vi "NI 5772 (AC) - Digitizer_v1.2 (FPGA).vi"() -> ()   [LabVIEW 2020]
doc: "Example Description:\nThis example demonstrates how to enable Time Interleaved Sampling with the NI 5772 adapter module to achieve a sampling rate of 1.6GS/s. This example continuously acquires records of analog input data from the NI 5772 adapter module. It allows you to select an AI channel, trigger type, and record size. This VI must be compiled before it is run. \n\nRunning the VI:\nThis VI must be run from the NI 5772 - Getting Started (Host).vi. Refer to the host VI documentation for steps regarding running and configuring the FPGA VI. \n\nExecution Steps:\nRefer to the Block Diagram of this VI for execution comments."
uses:
  Controls/AI Trigger Type.ctl
  Controls/Aquire State.ctl
  <vilib>/Platform/TimedLoop/XDataNode/timing_clust.ctl
  <vilib>/Platform/TimedLoop/XDataNode/nitl_modes.ctl
  <vilib>/Platform/TimedLoop/XDataNode/wakeup.ctl
  Controls/DigitizerState.ctl
  <vilib>/rvi/Emulation/niFpgaGetClockAttributes.vi
  <vilib>/rvi/Emulation/niFpgaSctlEmulationGetInTimedLoop.vi
  <vilib>/rvi/Emulation/niFpgaEmulationReportErrorSimple.vi
  <vilib>/rvi/eio/common/nirviEmuTemplateMethod_errors.vi
  <vilib>/rvi/Emulation/niFpgaCriticalErrorInLSC.vi
  <vilib>/rvi/Emulation/niFpgaProcessEmulError.vi
  <vilib>/rvi/Emulation/niFpgaEmulationIsFPGAContextNoSignature.vi
  <vilib>/rvi/errors/niFpgaSetErrorForExecOnDevCompSimple.vi
  <vilib>/rvi/eio/common/nirviEmuReportErrorAndStop.vi
  <vilib>/rvi/DataTransferAndStorage/Container/Common/niFpgaContainerGetUniqueNameForEmu.vi
  <vilib>/rvi/FIFO/Fifo_Resource/nirvififoEmulationSetSize.vi
  <vilib>/rvi/FIFO/Fifo_Resource/nirviFifoEmulationQueueMgr.vi
  <instcachedir>/0/nirviFifoEmulationQueueMgr_E5CAEC123FF24DC58D834DCA3CDAA9B5.lvgen/nirviFifoEmulationQueueMgr_E5CAEC123FF24DC58D834DCA3CDAA9B5_004.vi
  <vilib>/Utility/error.llb/Clear Errors.vi
  <vilib>/rvi/FIFO/Fifo_Resource/nirvififoEmulationCreateLock.vi
  <vilib>/rvi/FIFO/Fifo_Resource/nirvififoEmulationObtainLock.vi
  <vilib>/rvi/FIFO/Fifo_Resource/nirvififoEmulationReleaseLock.vi
  <vilib>/rvi/occurrence/nirviWaitOnOccurrenceBase.vi
  <vilib>/rvi/errors/nirviReportUnexpectedCaseInternalError.vi
  <vilib>/rvi/errors/nirviReportUnexpectedCaseInternalError (U32).vi
  <vilib>/rvi/Memory/Memory_Emulation/nirvimemoryFastEmulation.vi
  <vilib>/rvi/Memory/Memory_Emulation/nirvimemoryEmulation.vi
  <instcachedir>/0/nirviFifoEmulationQueueMgr_E5CAEC123FF24DC58D834DCA3CDAA9B5.lvgen/nirviFifoEmulationQueueMgr_E5CAEC123FF24DC58D834DCA3CDAA9B5_000.vi
  <vilib>/rvi/interface/RandomDataEmulation/niFpgaRandomDataHandleErrors.vi
  <vilib>/rvi/FIFO/Fifo_Resource/nirvififoEmulationDetermineInputValidOut.vi
  <instrlib>/_niInstr/Basic Elements/v1/FPGA/Private/Count Up U64.vi
  <vilib>/eio/EIONode/EIONode.xnode
  <vilib>/rvi/DataTransferAndStorage/Container/XNode/niFpgaContainer.xnode
  <vilib>/rvi/FIFO/Fifo_Resource/nirvififoEmulationRead.vi
  <vilib>/Platform/TimedLoop/XDataNode/XDataNode.xnode
  <vilib>/rvi/interface/RandomDataEmulation/nirviRandomDataFpgaReadWriteTemplate.vi
  <vilib>/rvi/FIFO/Fifo_Resource/nirvififoEmulationWrite.vi
  <vilib>/Platform/TimedLoop/XDataNode/XDNodeRunTimeDep.lvlib
  <instrlib>/_niInstr/Basic Elements/v1/FPGA/niInstr Basic Elements v1 FPGA.lvlib
  <vilib>/rvi/FIFO/Fifo_Resource/nirvififoEmulationGetNumberOfElementsToRead.vi
panel:
  out "WaitForWave\nCompletion":u16
  in  "Wave Sampling Rate":sgl
  in  "WaveSampleCount":sgl format="%#_13g"
  in  "Delay (us)":sgl
  in  "AvgCount_powerOf2":i16=1
  out "DMA FIFO Overflow?":bool caption="FIFO Overflow?"
  out "Removed\nElement":u64
  out "AvgCount":u16=1
  in  "vi/nGenTrig":bool
  in  "TrigIn Simulate":bool
  out "Trig Count":u64
  in  "Clear Count":bool
  out "Delay after Trig [cycles]":u16
  out "TS FIFO In Overflow?":bool caption="FIFO Overflow?"
  in  "Samples Per Trigger":u16=512 min=1 step=1
  in  "Arm Trigger":bool
  in  "User Command Commit":bool
  in  "User Command":u8
  out "User Command Idle":bool
  out "User Command Status":u8
  in  "User Data 0":u16
  in  "User Data 1":u8
  out "PLL Locked":bool
  out "User Error":bool
  out "Configured?":bool
  in  "Trigger Level":i16
  in  "Trigger Type":T1
  # "Resource Configuration"
  # "Analog Input"
  # "Clock Configuration"
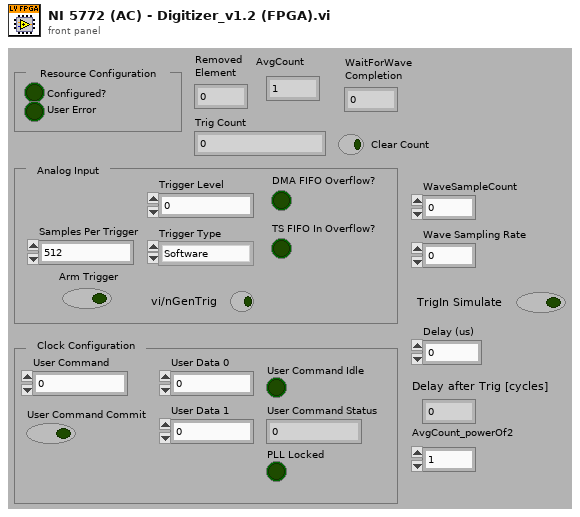
[diagram p1: front panel]
types:
  T1 = typedef "AI Trigger Type.ctl" = enum8{"Software", "Data Edge"}
  T2 = typedef "DigitizerState.ctl" = enum16{"Init", "Build/Clear Accumulator", "GetData", "AverageCountCheck", "SendtoHost"}
  T3 = typedef "Aquire State.ctl" = enum8{"Idle", "Wait for Trigger", "Hold Aquire", "Acquire", "WaitForWaveCompletion", "CheckAvg"}
  T4 = typedef "XDNodeRunTimeDep.lvlib/timing_clust.ctl" = cluster{"Expected End [f-1]":u64, "Actual End [f-1]":u64, "Finished Late? [f-1]":bool, "Expected End [i-1]":u64, "Actual End [i-1]":u64, "Finished Late? [i-1]":bool, "Expected Start [i]":u64, "Actual Start [i]":u64, "Expected Start [f]":u64, "Actual Start [f]":u64, "Source Name":string, "Structure Name":string, "Period":i64, "Deadline":i64, "Offset":i64, "Start":i64, "Priority":i32, "Timeout":i32, "Mode":T5, "Wakeup Reason":T6, "Error":errorcluster, "Source Type":string, "Secondary Source Type":string, "Global End Time":u64, "Global Start Time":u64, "Frame Duration":u64, "Iteration Duration":u64, "Assigned CPU":i32, "I/O Scan Engine Mode":u32}
  T5 = typedef "XDNodeRunTimeDep.lvlib/nitl_modes.ctl" = enum32{"No Change", "Process missed periods, maintain original phase", "Discard missed periods, maintain original phase", "Process missed periods, ignore original phase", "Discard missed periods, ignore original phase"}
  T6 = typedef "XDNodeRunTimeDep.lvlib/wakeup.ctl" = enum32{"Normal", "Aborted", "Asynchronous wakeup", "Timing source error", "Timed loop error", "Timeout"}
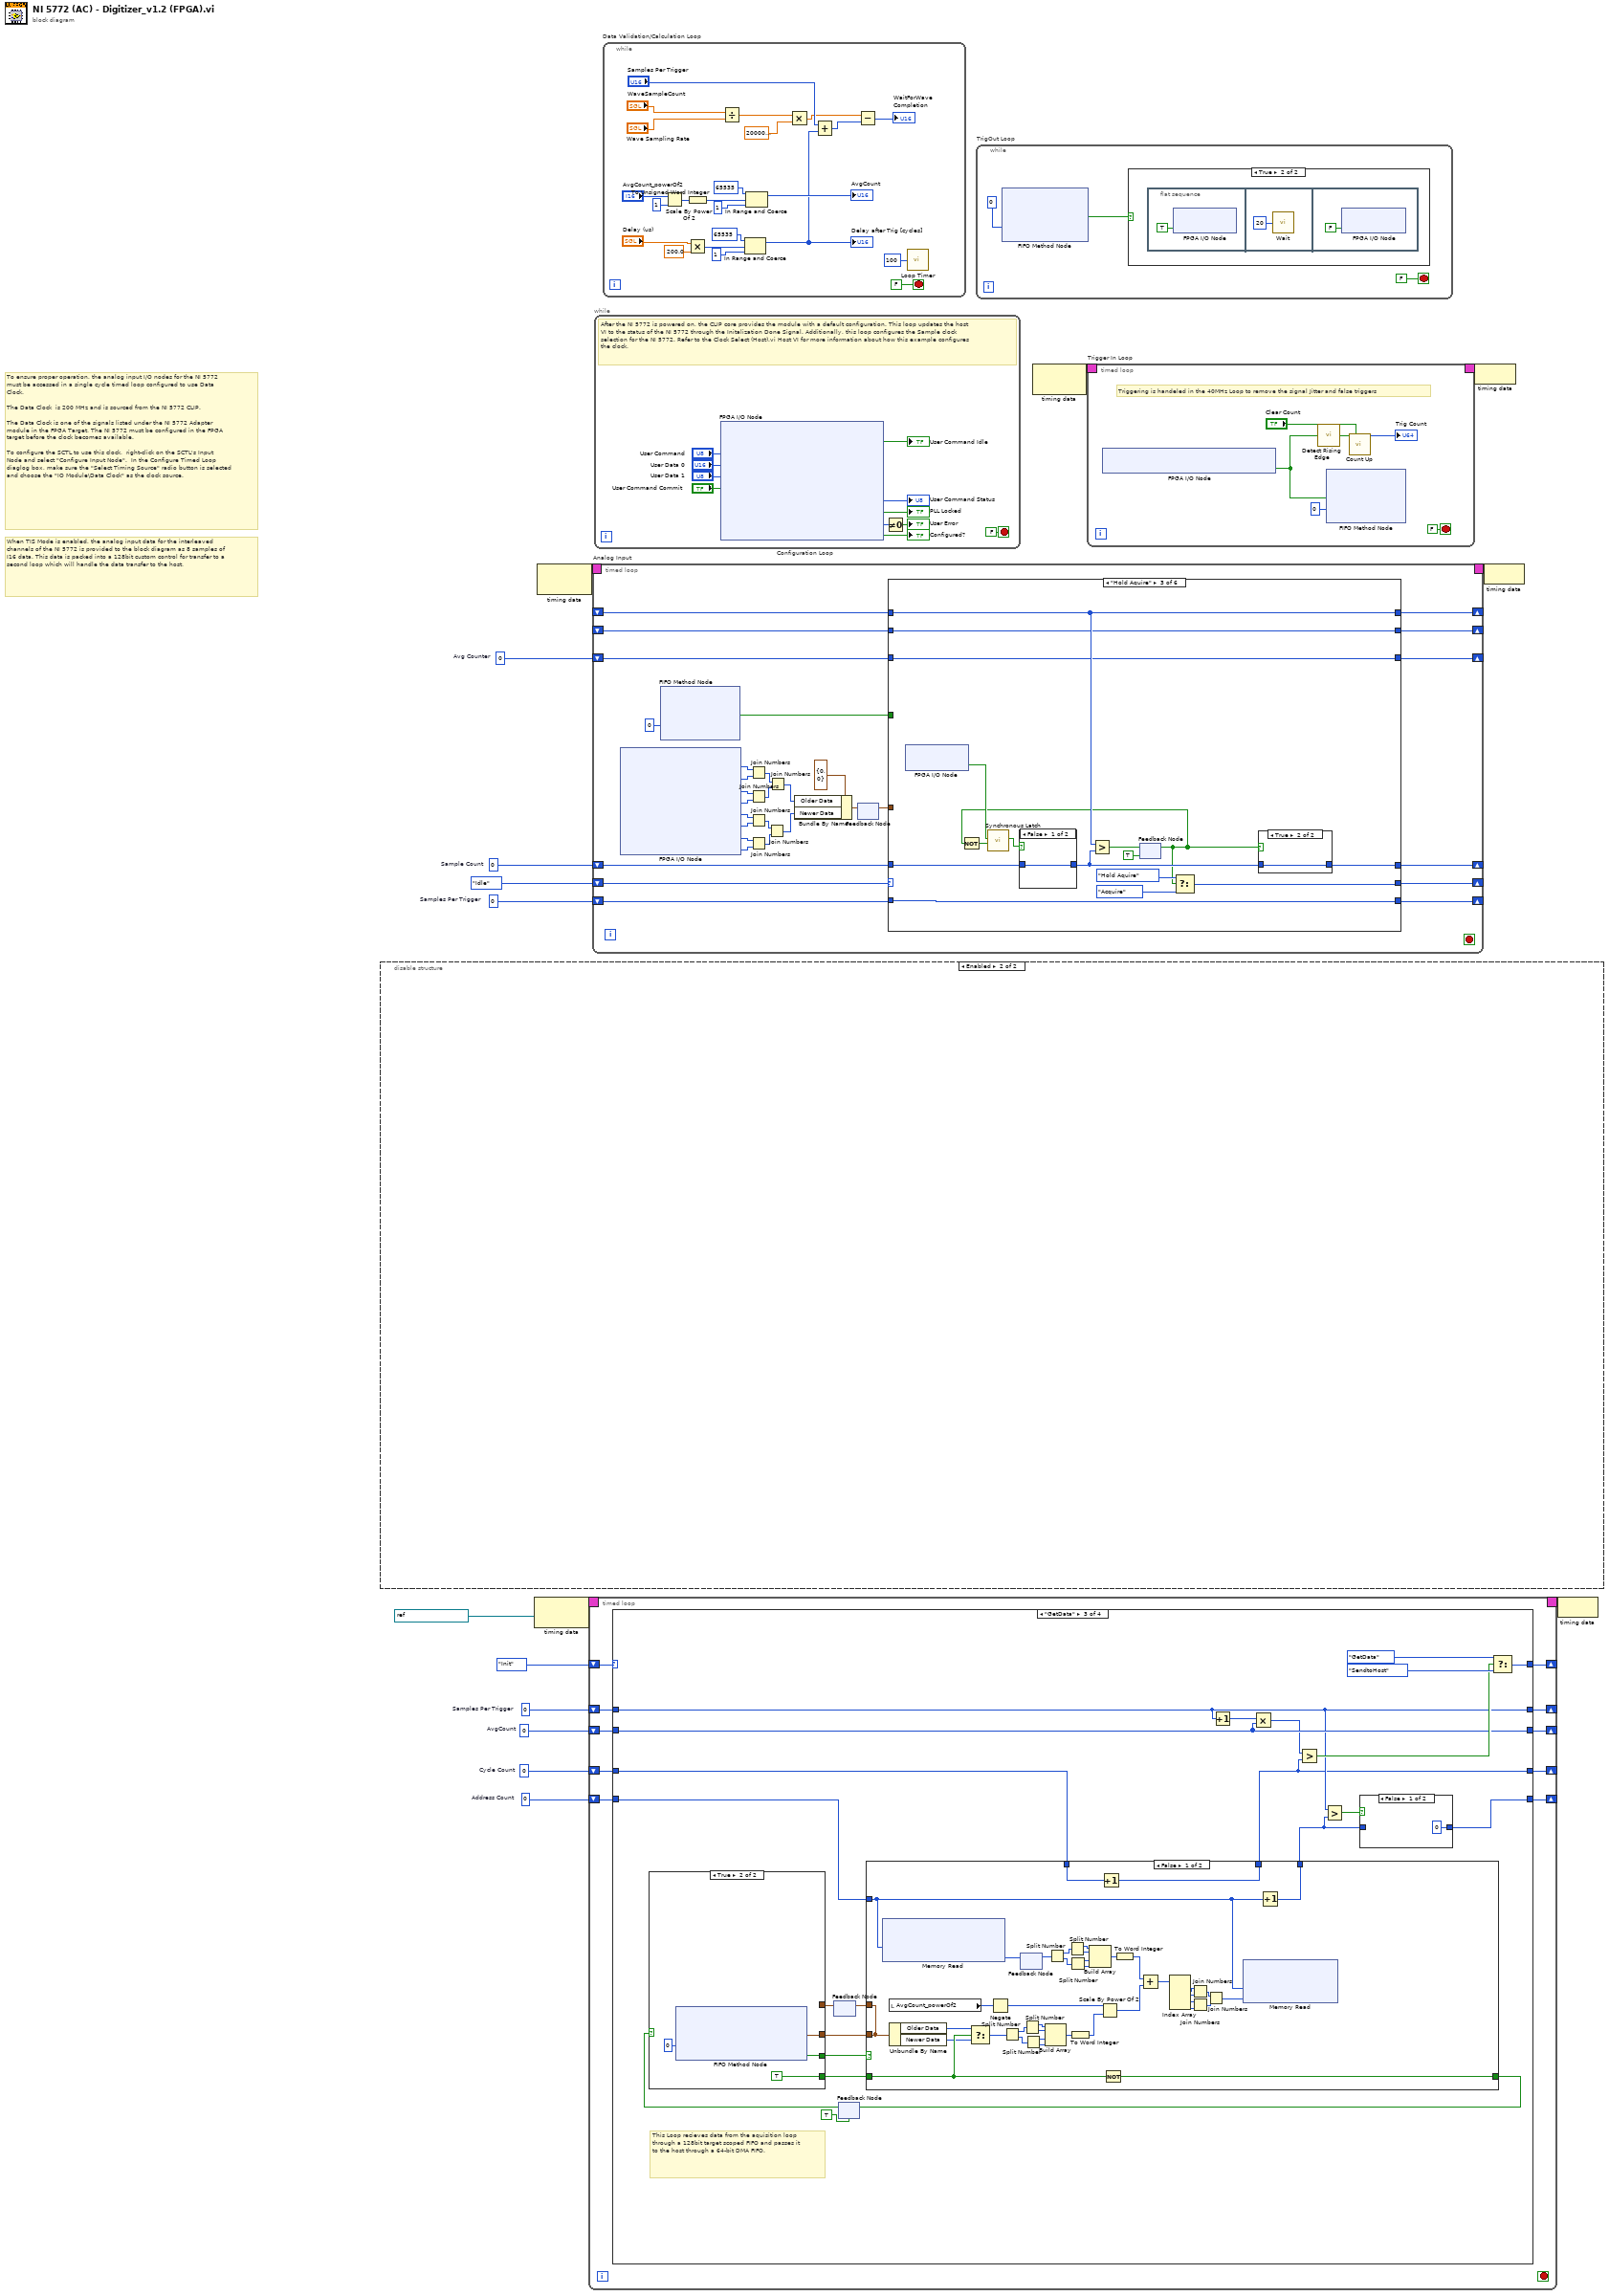
[diagram p0: block diagram]
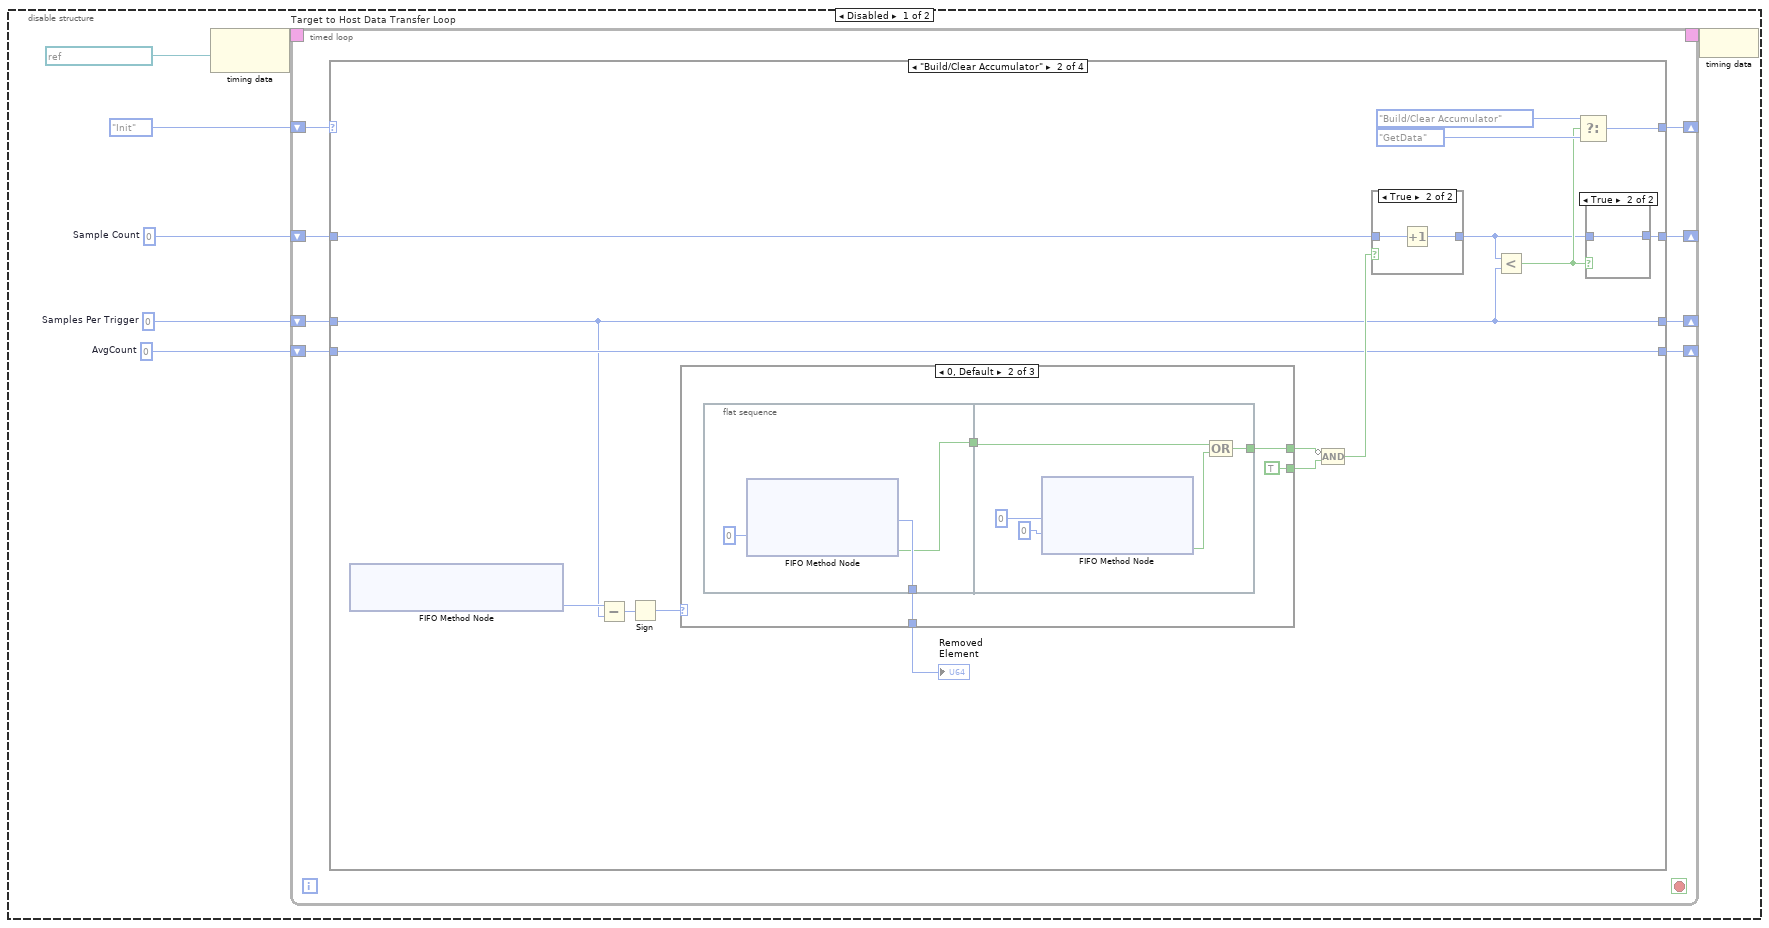
[diagram p2: hidden frame]
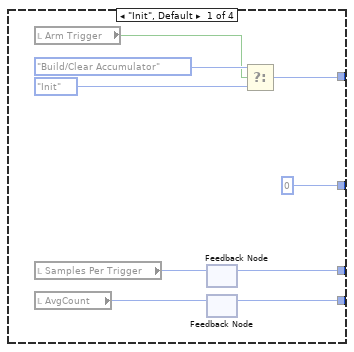
[diagram p3: hidden frame]
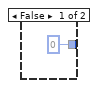
[diagram p4: hidden frame]
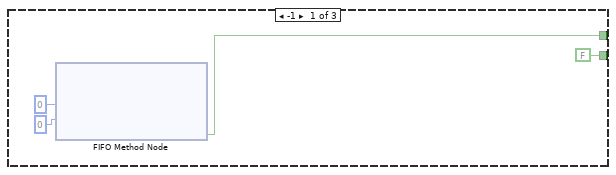
[diagram p6: hidden frame]
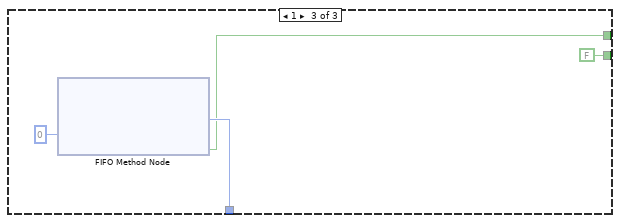
[diagram p7: hidden frame]
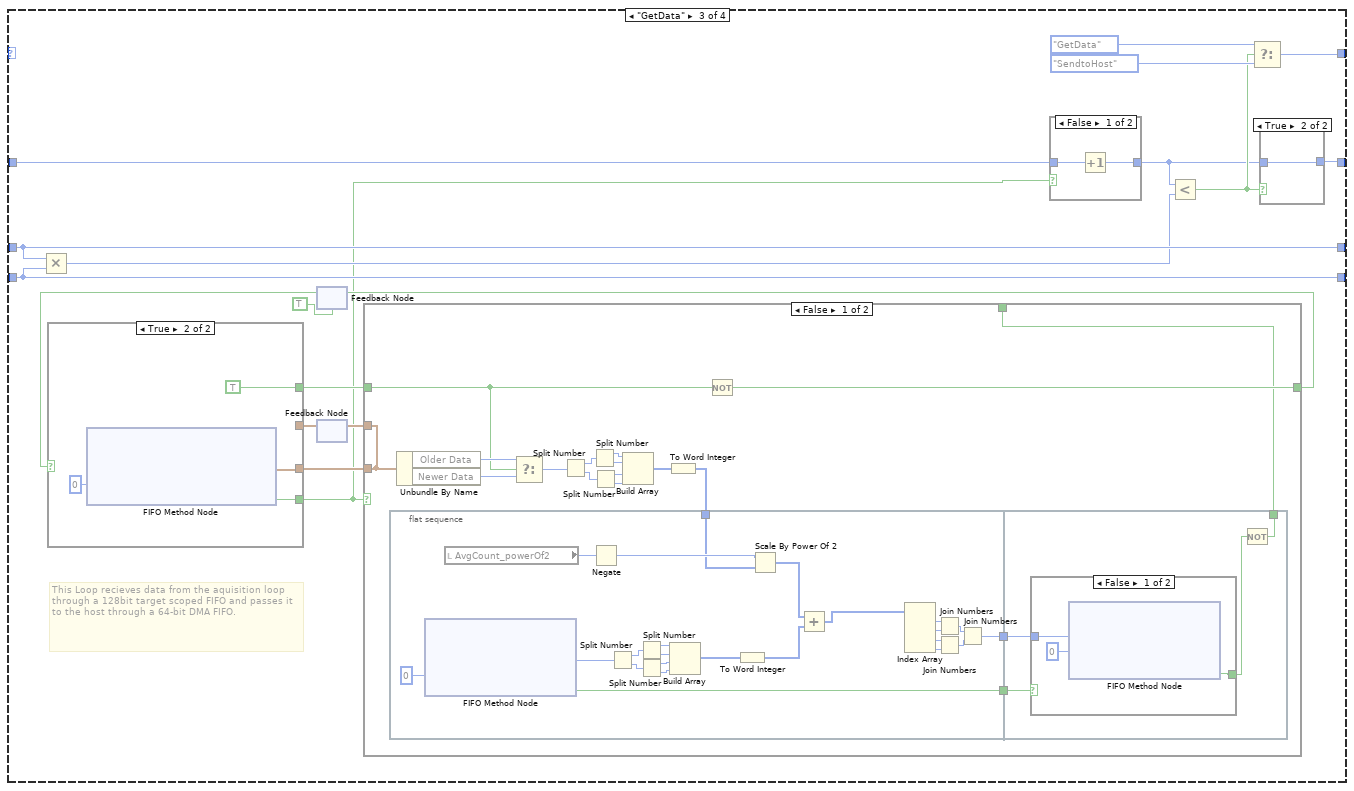
[diagram p8: hidden frame]
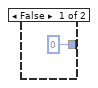
[diagram p9: hidden frame]
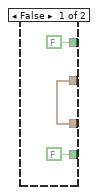
[diagram p11: hidden frame]
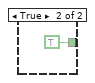
[diagram p12: hidden frame]
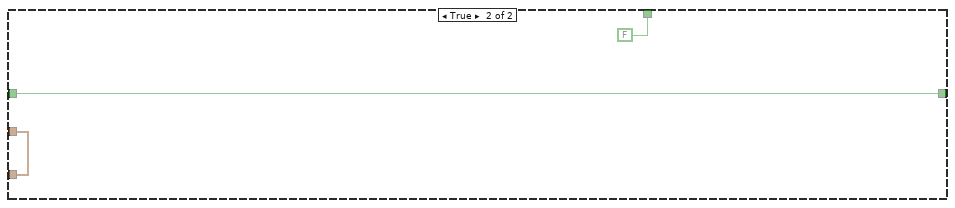
[diagram p13: hidden frame]
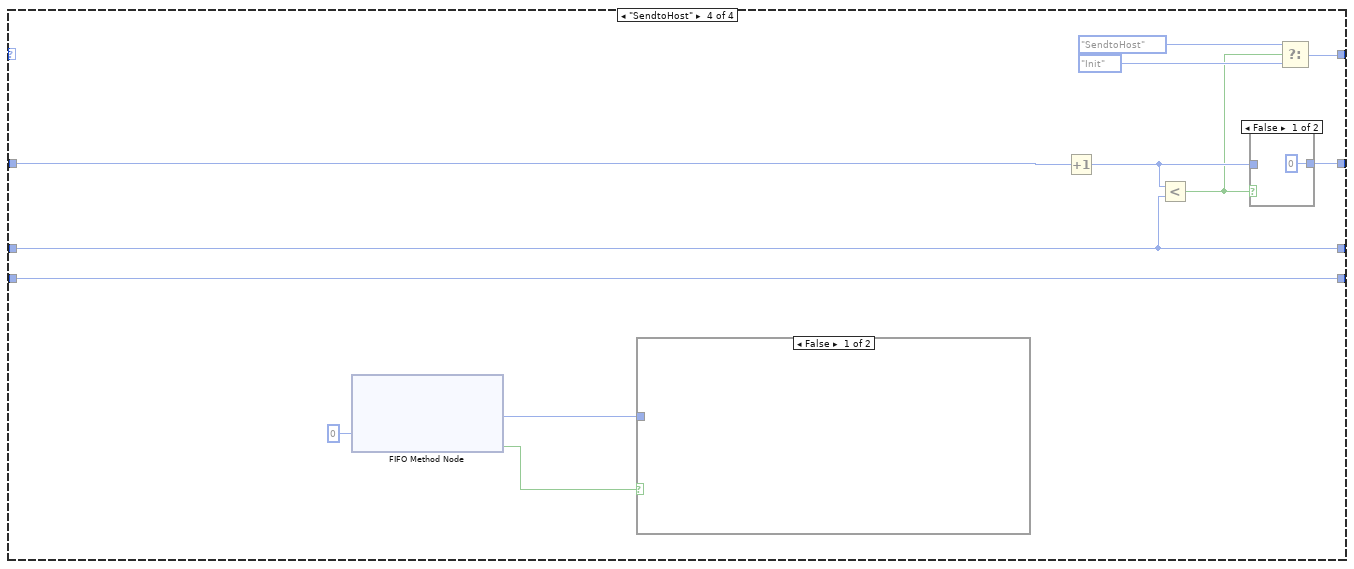
[diagram p14: hidden frame]
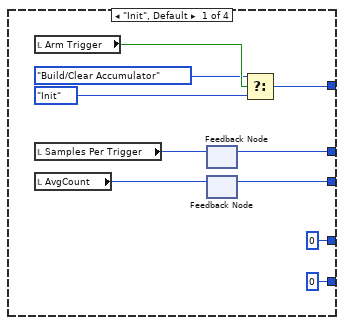
[diagram p17: hidden frame]
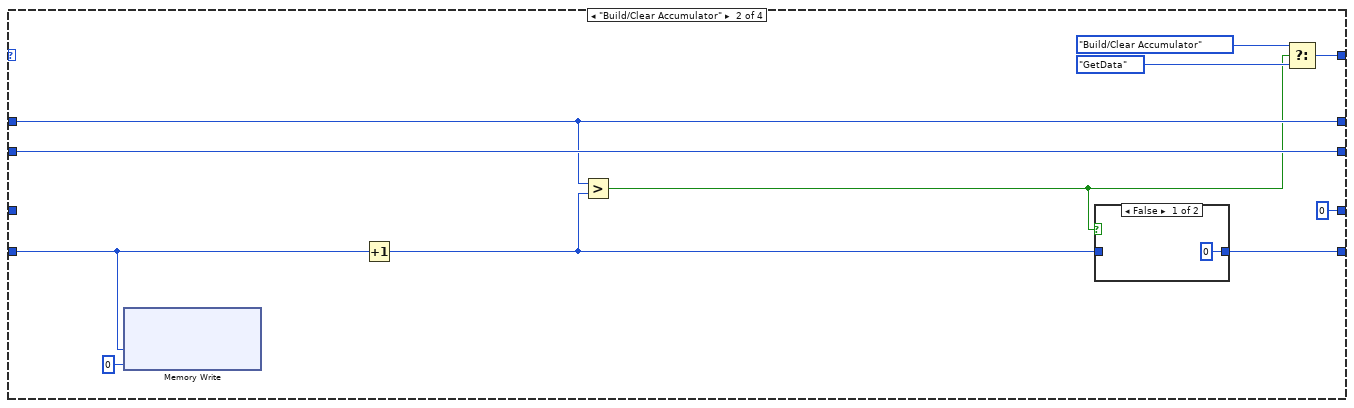
[diagram p18: hidden frame]
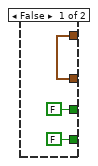
[diagram p20: hidden frame]
diagram:
  w1 = u32 0  # Cycle Count
  w2 = u32 0  # Address Count
  w3 = u16 0  # AvgCount
  w4 = u16 0  # Samples Per Trigger
  w9 = u16 0  # Avg Counter
  w12 = u16 0  # Samples Per Trigger
  w13 = u16 0  # Sample Count
  # "When TIS Mode is enabled, the analog input data for the interleaved channels of the NI 5772 is provided to the block diagram as 8 samples of I16 data. This data is packed into a 128bit custom control for transfer to a second loop which will handle the data transfer to the host."
  # "To ensure proper operation, the analog input I/O nodes for the NI 5772 must be accessed in a single cycle timed loop configured to use Data Clock. \n\nThe Data Clock  is 200 MHz and is sourced from the NI 5772 CLIP.\n\nThe Data Clock is one of the signals listed under the NI 5772 Adapter module in the FPGA Target. The NI 5772 must be configured in the FPGA target before the clock becomes available. \n\nTo configure the SCTL to use this clock,  right-click on the SCTL's Input Node and select \"Configure Input Node\".  In the Configure Timed Loop diaglog box, make sure the \"Select Timing Source\" radio button is selected and choose the \"IO Module\\Data Clock\" as the clock source."
  n1 = disable-structure shown="Enabled" {
    frame Disabled {
      w17 = u16 0  # Sample Count
      w18 = u16 0  # Samples Per Trigger
      w19 = u16 0  # AvgCount
      n2 = node-c288(refnum<k21> "100 MHz Clock" ("Source Name")) -> (w23:T4)
      n3 = timed-loop "Target to Host Data Transfer Loop" {
        timing: w23 -> [_]
        timing-out: [_] -> w22
        shift-right: [w26] -> _
        shift-left: DigitizerState."Init" -> [w31]
        shift-right: [w30] -> _
        shift-left: w18 -> [w29]
        shift-right: [w28] -> _
        shift-left: w19 -> [w27]
        shift-right: [w24] -> _
        shift-left: w17 -> [w25]
        stop <- _ stop-if-true
        n4 = case shown="\"Build/Clear Accumulator\"" w31 {
          tunnel: [w39 w44 w92 w166] -> w30
          tunnel: w29 -> [_ w44 w92 w166]
          tunnel: [w37 w45 w91 w173] -> w28
          tunnel: w27 -> [_ w45 w91 w173]
          tunnel: [w33 w52 w86 w169] -> w26
          tunnel: w25 -> [_ w47 w85 w167]
          tunnel: [u16 0 ("Sample Count") w41 w84 w164] -> w24
          frame "Init", Default {
            n5 = local read "Arm Trigger"() -> (w34:bool)
            n6 = local read "Samples Per Trigger"() -> (w40:u16)
            n7 = local read "AvgCount"() -> (w38:u16)
            n8 = feedback #1() -> (w39:u16)  [unwired: 1 in]
            n9 = feedback-in #1(w40) -> ()
            n10 = feedback #2() -> (w37:u16)  [unwired: 1 in]
            n11 = feedback-in #2(w38) -> ()
            n12 = Select(t=DigitizerState."Build/Clear Accumulator", s=w34, f=DigitizerState."Init") -> (s? t:f=w33:T2)
          }
          frame "Build/Clear Accumulator" {
            n13 = xnode ("FIFO Method Node")() -> ("Number of Elements to Read"=w56:u32)  [unwired: 1 in, 1 out]
            n14 = Subtract(x=w56, y=w44) -> (x-y=w55:i8)
            n15 = Sign(1:w55) -> (0:w54:i8)
            n16 = case shown="0, Default" w54 {
              tunnel: [_ w69 w80] -> w53
              tunnel: [w63 w67 w79] -> w49
              tunnel: [FALSE TRUE FALSE] -> w48
              frame -1 {
                n17 = xnode ("FIFO Method Node")("Element"=u64 0, "Timeout"=0) -> ("Timed Out?"=w63:bool)  [unwired: 1 in, 1 out]
              }
              frame 0, Default {
                n18 = flat-sequence {
                  tunnel: [w71] -> w69
                  tunnel: [w70] -> w68
                  tunnel: w68 -> [w75]
                  tunnel: [w73] -> w67
                  frame #0 {
                    n19 = xnode ("FIFO Method Node")("Timeout"=0) -> ("Element"=w71:u64, "Timed Out?"=w70:bool)  [unwired: 1 in, 1 out]
                  }
                  frame #1 {
                    n20 = xnode ("FIFO Method Node")("Element"=u64 0 ("y"), "Timeout"=0) -> ("Timed Out?"=w74:bool)  [unwired: 1 in, 1 out]
                    n21 = Compound Arithmetic op=OR(w75, w74) -> (w73:bool)
                  }
                }
              }
              frame 1 {
                n22 = xnode ("FIFO Method Node")("Timeout"=0) -> ("Element"=w80:u64, "Timed Out?"=w79:bool)  [unwired: 1 in, 1 out]
              }
            }
            "Removed\nElement" <- w53
            n23 = Compound Arithmetic op=AND(invert w49, w48) -> (w46:bool)
            n24 = case shown="True" w46 {
              tunnel: w47 -> [w59 w61]
              tunnel: [w59 w60] -> w42
              frame False {
              }
              frame True {
                n25 = Increment(x=w61) -> (x+1=w60:u16)
              }
            }
            n26 = Less?(x=w42, y=w44) -> (x < y?=w43:bool)
            n27 = Select(t=DigitizerState."Build/Clear Accumulator", s=w43, f=DigitizerState."GetData") -> (s? t:f=w52:T2)
            n28 = case shown="True" w43 {
              tunnel: [u16 0 ("Sample Count") w58] -> w41
              tunnel: w42 -> [_ w58]
              frame False {
              }
              frame True {
              }
            }
          }
          frame "GetData" {
            # "This Loop recieves data from the aquisition loop through a 128bit target scoped FIFO and passes it to the host through a 64-bit DMA FIFO."
            n29 = Multiply(x=w92, y=w91) -> (x*y=w83:u16)
            n30 = feedback #3(TRUE ("Timed Out?")) -> (w97:bool)
            n31 = feedback #4() -> (w96:cluster{"Older Data":u64, "Newer Data":u64})  [unwired: 1 in]
            n32 = case shown="True" w97 {
              tunnel: [w105 w108] -> w94
              tunnel: [FALSE ("Timed Out?") w109] -> w82
              tunnel: [FALSE ("Timed Out?") TRUE ("Timed Out?")] -> w93
              tunnel: w96 -> [w105 _]
              frame False {
              }
              frame True {
                n33 = xnode ("FIFO Method Node")("Timeout"=0) -> ("Element"=w108:cluster{"Older Data":u64, "Newer Data":u64}, "Timed Out?"=w109:bool)  [unwired: 1 in, 1 out]
              }
            }
            n34 = case shown="False" w82 {
              tunnel: [w126 w162] -> w98
              tunnel: w93 -> [w127 w162]
              tunnel: w94 -> [w125 w161]
              tunnel: [w125 w161] -> w95
              tunnel: [w113 FALSE ("increment")] -> _
              frame False {
                n35 = flat-sequence {
                  tunnel: [w129] -> w117
                  tunnel: [w140] -> w115
                  tunnel: w112 -> [w136]
                  tunnel: w117 -> [w155]
                  tunnel: [w152] -> w113
                  tunnel: w115 -> [w154]
                  frame #0 {
                    n36 = xnode ("FIFO Method Node")("Timeout"=0) -> ("Element"=w139:u64, "Timed Out?"=w140:bool)  [unwired: 1 in, 1 out]
                    n37 = local read "AvgCount_powerOf2"() -> (w138:i16)
                    n38 = Negate(x=w138) -> (-x=w137:i16)
                    n39 = Split Number(x=w139) -> (hi(x)=w145:u32, lo(x)=w146:u32)
                    n40 = Split Number(x=w145) -> (hi(x)=w147:u16, lo(x)=w148:u16)
                    n41 = Split Number(x=w146) -> (hi(x)=w149:u16, lo(x)=w150:u16)
                    n42 = Build Array(w147, w148, w149, w150) -> (w151:u16[])
                    n43 = To Word Integer(number=w151) -> (16bit integer=w143:i16[])
                    n44 = Scale By Power Of 2(n=w137, x=w136) -> (x*2^n=w135:i16[])
                    n45 = Add(x=w135, y=w143) -> (x+y=w134:i16[])
                    n46 = Index Array(array=w134) -> (element #1=w133:i16, element #2=w132:i16, element #3=w131:i16, element #4=w130:i16)  [unwired: 4 in]
                    n47 = Join Numbers(hi=w133, lo=w132) -> ((hi.lo)=w142:u32)
                    n48 = Join Numbers(hi=w131, lo=w130) -> ((hi.lo)=w141:u32)
                    n49 = Join Numbers(hi=w142, lo=w141) -> ((hi.lo)=w129:u64)
                  }
                  frame #1 {
                    n50 = case shown="False" w154 {
                      tunnel: w155 -> [w157 _]
                      tunnel: [w156 TRUE ("Timed Out?")] -> w153
                      frame False {
                        n51 = xnode ("FIFO Method Node")("Element"=w157, "Timeout"=0) -> ("Timed Out?"=w156:bool)  [unwired: 1 in, 1 out]
                      }
                      frame True {
                      }
                    }
                    n52 = Not(x=w153) -> (.not. x?=w152:bool)
                  }
                }
                n53 = Unbundle By Name(w125) -> ("Older Data"=w128:u64, "Newer Data"=w124:u64)
                n54 = Select(t=w128, s=w127, f=w124) -> (s? t:f=w114:u64)
                n55 = Split Number(x=w114) -> (hi(x)=w118:u32, lo(x)=w119:u32)
                n56 = Split Number(x=w118) -> (hi(x)=w120:u16, lo(x)=w121:u16)
                n57 = Split Number(x=w119) -> (hi(x)=w122:u16, lo(x)=w123:u16)
                n58 = Build Array(w120, w121, w122, w123) -> (w116:u16[])
                n59 = To Word Integer(number=w116) -> (16bit integer=w112:i16[])
                n60 = Not(x=w127) -> (.not. x?=w126:bool)
              }
              frame True {
              }
            }
            n61 = feedback-in #3(w98) -> ()
            n62 = feedback-in #4(w95) -> ()
            n63 = case shown="False" w82 {
              tunnel: w85 -> [w103 w104]
              tunnel: [w102 w104] -> w87
              frame False {
                n64 = Increment(x=w103) -> (x+1=w102:u16)
              }
              frame True {
              }
            }
            n65 = Less?(x=w87, y=w83) -> (x < y?=w88:bool)
            n66 = Select(t=DigitizerState."GetData", s=w88, f=DigitizerState."SendtoHost") -> (s? t:f=w86:T2)
            n67 = case shown="True" w88 {
              tunnel: [u16 0 ("Sample Count") w101] -> w84
              tunnel: w87 -> [_ w101]
              frame False {
              }
              frame True {
              }
            }
          }
          frame "SendtoHost" {
            n68 = xnode ("FIFO Method Node")("Timeout"=0) -> ("Element"=w172:u64, "Timed Out?"=w163:bool)  [unwired: 1 in, 1 out]
            n69 = case shown="False" w163 {
              tunnel: w172 -> [_ _]
              frame False {
              }
              frame True {
              }
            }
            n70 = Increment(x=w167) -> (x+1=w168:u16)
            n71 = Less?(x=w168, y=w166) -> (x < y?=w165:bool)
            n72 = case shown="False" w165 {
              tunnel: [u16 0 ("Sample Count") w176] -> w164
              tunnel: w168 -> [_ w176]
              frame False {
              }
              frame True {
              }
            }
            n73 = Select(t=DigitizerState."SendtoHost", s=w165, f=DigitizerState."Init") -> (s? t:f=w169:T2)
          }
        }
      }
      n74 = node-c288(w22) -> ()
    }
    frame Enabled {
    }
  }
  n75 = node-c288(refnum<k21> "100 MHz Clock" ("Source Name")) -> (w8:T4)
  n76 = node-c288() -> (w16:T4)  [unwired: 1 in]
  n77 = timed-loop {
    timing: w8 -> [_]
    timing-out: [_] -> w7
    shift-right: [w191] -> _
    shift-left: DigitizerState."Init" -> [w192]
    shift-right: [w190] -> _
    shift-left: w4 -> [w188]
    shift-right: [w189] -> _
    shift-left: w3 -> [w187]
    shift-right: [w185] -> _
    shift-left: w2 -> [w186]
    shift-right: [w183] -> _
    shift-left: w1 -> [w184]
    stop <- _ stop-if-true
    n78 = case shown="\"GetData\"" w192 {
      tunnel: [w197 w207 w235 w302] -> w191
      tunnel: [w196 w210 w218 w305] -> w190
      tunnel: [w195 w211 w224 w306] -> w189
      tunnel: w188 -> [_ w210 w218 w305]
      tunnel: w187 -> [_ w211 w224 w306]
      tunnel: w186 -> [_ w213 w221 w307]
      tunnel: [u32 0 w204 w233 w299] -> w185
      tunnel: w184 -> [_ _ w217 _]
      tunnel: [u32 0 ("Cycle Count") u32 0 ("Cycle Count") w216 u32 0 ("Cycle Count")] -> w183
      frame "Init", Default {
        n79 = local read "Arm Trigger"() -> (w202:bool)
        n80 = local read "Samples Per Trigger"() -> (w198:u16)
        n81 = local read "AvgCount"() -> (w199:u16)
        n82 = feedback #5() -> (w196:u16)  [unwired: 1 in]
        n83 = feedback-in #5(w198) -> ()
        n84 = feedback #6() -> (w195:u16)  [unwired: 1 in]
        n85 = feedback-in #6(w199) -> ()
        n86 = Select(t=DigitizerState."Build/Clear Accumulator", s=w202, f=DigitizerState."Init") -> (s? t:f=w197:T2)
      }
      frame "Build/Clear Accumulator" {
        n87 = xnode "Memory Write"("Address"=w213, "Data"=u64 0) -> ()  [unwired: 1 in, 1 out]
        n88 = Increment(x=w213) -> (x+1=w205:u32)
        n89 = Greater?(x=w210, y=w205) -> (0:w206:bool)
        n90 = case shown="False" w206 {
          tunnel: w205 -> [_ w215]
          tunnel: [u32 0 w215] -> w204
          frame False {
          }
          frame True {
          }
        }
        n91 = Select(t=DigitizerState."Build/Clear Accumulator", s=w206, f=DigitizerState."GetData") -> (s? t:f=w207:T2)
      }
      frame "GetData" {
        # "This Loop recieves data from the aquisition loop through a 128bit target scoped FIFO and passes it to the host through a 64-bit DMA FIFO."
        n92 = feedback #7() -> (w228:cluster{"Older Data":u64, "Newer Data":u64})  [unwired: 1 in]
        n93 = feedback #8(TRUE ("Timed Out?")) -> (w227:bool)
        n94 = case shown="True" w227 {
          tunnel: [w238 w241] -> w230
          tunnel: [FALSE ("Timed Out?") w242] -> w232
          tunnel: [FALSE ("Timed Out?") TRUE ("Timed Out?")] -> w231
          tunnel: w228 -> [w238 _]
          frame False {
          }
          frame True {
            n95 = xnode ("FIFO Method Node")("Timeout"=0) -> ("Element"=w241:cluster{"Older Data":u64, "Newer Data":u64}, "Timed Out?"=w242:bool)  [unwired: 1 in, 1 out]
          }
        }
        n96 = case shown="False" w232 {
          tunnel: [w281 w287] -> w226
          tunnel: w231 -> [w282 w287]
          tunnel: w230 -> [w280 w286]
          tunnel: [w280 w286] -> w229
          tunnel: w221 -> [w257 w285]
          tunnel: [w270 w285] -> w220
          tunnel: w217 -> [w246 w284]
          tunnel: [w245 w284] -> w216
          frame False {
            n97 = xnode "Memory Read"("Address"=w257) -> ("Data"=w248:u64)  [unwired: 1 in, 1 out]
            n98 = local read "AvgCount_powerOf2"() -> (w261:i16)
            n99 = Unbundle By Name(w280) -> ("Older Data"=w283:u64, "Newer Data"=w279:u64)
            n100 = Select(t=w283, s=w282, f=w279) -> (s? t:f=w271:u64)
            n101 = Negate(x=w261) -> (-x=w262:i16)
            n102 = Split Number(x=w271) -> (hi(x)=w273:u32, lo(x)=w274:u32)
            n103 = feedback-in #9(w248) -> ()
            n104 = feedback #9() -> (w247:u64)  [unwired: 1 in]
            n105 = Split Number(x=w273) -> (hi(x)=w275:u16, lo(x)=w276:u16)
            n106 = Split Number(x=w274) -> (hi(x)=w277:u16, lo(x)=w278:u16)
            n107 = Build Array(w275, w276, w277, w278) -> (w272:u16[])
            n108 = Split Number(x=w247) -> (hi(x)=w269:u32, lo(x)=w268:u32)
            n109 = Split Number(x=w269) -> (hi(x)=w267:u16, lo(x)=w266:u16)
            n110 = Split Number(x=w268) -> (hi(x)=w265:u16, lo(x)=w264:u16)
            n111 = To Word Integer(number=w272) -> (16bit integer=w260:i16[])
            n112 = Build Array(w267, w266, w265, w264) -> (w263:u16[])
            n113 = Scale By Power Of 2(n=w262, x=w260) -> (x*2^n=w259:i16[])
            n114 = Increment(x=w246) -> (x+1=w245:u32)
            n115 = Not(x=w282) -> (.not. x?=w281:bool)
            n116 = To Word Integer(number=w263) -> (16bit integer=w258:i16[])
            n117 = Add(x=w258, y=w259) -> (x+y=w250:i16[])
            n118 = Index Array(array=w250) -> (element #1=w253:i16, element #2=w254:i16, element #3=w255:i16, element #4=w256:i16)  [unwired: 4 in]
            n119 = Join Numbers(hi=w253, lo=w254) -> ((hi.lo)=w251:u32)
            n120 = Join Numbers(hi=w255, lo=w256) -> ((hi.lo)=w252:u32)
            n121 = Join Numbers(hi=w251, lo=w252) -> ((hi.lo)=w249:u64)
            n122 = xnode "Memory Read"("Address"=w257, "Data"=w249) -> ()  [unwired: 1 in, 1 out]
            n123 = Increment(x=w257) -> (x+1=w270:u32)
          }
          frame True {
          }
        }
        n124 = feedback-in #7(w229) -> ()
        n125 = feedback-in #8(w226) -> ()
        n126 = Increment(x=w218) -> (x+1=w219:u16)
        n127 = Multiply(x=w219, y=w224) -> (x*y=w223:u16)
        n128 = Greater?(x=w223, y=w216) -> (0:w234:bool)
        n129 = Greater?(x=w218, y=w220) -> (0:w222:bool)
        n130 = case shown="False" w222 {
          tunnel: w220 -> [_ w289]
          tunnel: [u32 0 w289] -> w233
          frame False {
          }
          frame True {
          }
        }
        n131 = Select(t=DigitizerState."GetData", s=w234, f=DigitizerState."SendtoHost") -> (s? t:f=w235:T2)
      }
      frame "SendtoHost" {
        # "Monitor for any DMA FIFO timeouts"
        n132 = xnode "Memory Write"("Address"=w307) -> ("Data"=w293:u64)  [unwired: 1 in, 1 out]
        n133 = feedback-in #10(w293) -> ()
        n134 = feedback #10() -> (w292:u64)  [unwired: 1 in]
        n135 = Increment(x=w307) -> (x+1=w300:u32)
        n136 = xnode ("FIFO Method Node")("Element"=w292, "Timeout"=0) -> ("Timed Out?"=w297:bool)  [unwired: 1 in, 1 out]
        n137 = Increment(x=w305) -> (x+1=w291:u16)
        n138 = feedback #11(FALSE) -> (w296:bool)
        n139 = Compound Arithmetic op=OR(w296, w297) -> (w298:bool)
        "DMA FIFO Overflow?" <- w298
        n140 = feedback-in #11(w298) -> ()
        n141 = Greater?(x=w291, y=w300) -> (0:w301:bool)
        n142 = case shown="False" w301 {
          tunnel: w300 -> [_ w309]
          tunnel: [u32 0 w309] -> w299
          frame False {
          }
          frame True {
          }
        }
        n143 = Select(t=DigitizerState."SendtoHost", s=w301, f=DigitizerState."Init") -> (s? t:f=w302:T2)
      }
    }
  }
  n144 = timed-loop "Analog Input" {
    timing: w16 -> [_]
    timing-out: [_] -> w15
    shift-right: [w341] -> _
    shift-left: Aquire_State."Idle" ("Acquire State") -> [w331]
    shift-right: [w342] -> _
    shift-left: w13 -> [w332]
    shift-right: [w340] -> _
    shift-left: w12 -> [w330]
    shift-right: [w317] -> _
    shift-left: _ -> [w316]
    shift-right: [w315] -> _
    shift-left: _ -> [w314]
    shift-right: [w312] -> _
    shift-left: w9 -> [w313]
    stop <- _ stop-if-true
    n145 = xnode "FPGA I/O Node"() -> ("IO Module\\AI 1 Data N-3"=w323:i16, "IO Module\\AI 0 Data N-3"=w322:i16, "IO Module\\AI 1 Data N-2"=w321:i16, "IO Module\\AI 0 Data N-2"=w320:i16, "IO Module\\AI 1 Data N-1"=w324:i16, "IO Module\\AI 0 Data N-1"=w325:i16, "IO Module\\AI 1 Data N"=w326:i16, "IO Module\\AI 0 Data N"=w327:i16)  [unwired: 8 in, 8 out]
    n146 = xnode ("FIFO Method Node")("Timeout"=0) -> ("Element"=w318:bool)  [unwired: 1 in, 2 out]
    n147 = Join Numbers(hi=w323, lo=w322) -> ((hi.lo)=w335:u32)
    n148 = Join Numbers(hi=w321, lo=w320) -> ((hi.lo)=w337:u32)
    n149 = Join Numbers(hi=w324, lo=w325) -> ((hi.lo)=w336:u32)
    n150 = Join Numbers(hi=w326, lo=w327) -> ((hi.lo)=w338:u32)
    n151 = Join Numbers(hi=w336, lo=w338) -> ((hi.lo)=w328:u64)
    n152 = Join Numbers(hi=w335, lo=w337) -> ((hi.lo)=w329:u64)
    n153 = Bundle By Name(cluster=cluster{"Older Data":u64, "Newer Data":u64} {"Older Data"=0, "Newer Data"=0} ("Element"), "Older Data"=w329, "Newer Data"=w328) -> (w333:cluster{"Older Data":u64, "Newer Data":u64})
    n154 = feedback #12() -> (w339:cluster{"Older Data":u64, "Newer Data":u64})  [unwired: 1 in]
    n155 = feedback-in #12(w333) -> ()
    n156 = case shown="\"Hold Aquire\"" w331 {
      tunnel: [u16 0 u16 0 w405 w416 w441 u16 0] -> w342
      tunnel: w332 -> [_ _ w404 w431 w440 _]
      tunnel: [w352 w364 w408 w430 w444 w455] -> w341
      tunnel: [w349 w368 w406 w427 w442 w453] -> w340
      tunnel: w330 -> [_ w368 w406 w427 w442 w453]
      tunnel: w339 -> [_ w367 _ w426 _ _]
      tunnel: w318 -> [_ w362 _ _ _ _]
      tunnel: [w347 w360 w403 w420 w439 w452] -> w317
      tunnel: w316 -> [_ w360 w403 w420 w439 w452]
      tunnel: [w345 w359 w401 w419 w436 w450] -> w315
      tunnel: w314 -> [_ w359 w401 w419 w436 w450]
      tunnel: [u16 0 ("Avg Count") w358 w400 w418 w435 w449] -> w312
      tunnel: w313 -> [_ w358 w400 w418 w435 w451]
      frame "Idle", Default {
        # "This state will wait for the host VI to arm the trigger."
        n157 = feedback-in #13("Arm Trigger") -> ()
        n158 = feedback #13() -> (w350:bool)  [unwired: 1 in]
        n159 = Select(t=Aquire_State."Wait for Trigger" ("Acquire State"), s=w350, f=Aquire_State."Idle" ("Acquire State")) -> (s? t:f=w352:T3)
        n160 = local read "Delay after Trig [cycles]"() -> (w348:u16)
        n161 = local read "AvgCount"() -> (w346:u16)
        n162 = local read "Samples Per Trigger"() -> (w343:u16)
        n163 = feedback #14() -> (w347:u16)  [unwired: 1 in]
        n164 = feedback-in #14(w348) -> ()
        n165 = feedback #15() -> (w345:u16)  [unwired: 1 in]
        n166 = feedback-in #15(w346) -> ()
        n167 = feedback-in #16(w343) -> ()
        n168 = feedback #16() -> (w349:u16)  [unwired: 1 in]
      }
      frame "Wait for Trigger" {
        # "After the trigger is armed, this state monitors for the specific trigger condition to begin the acquisition."
        n169 = feedback-in #17("Trigger Type") -> ()
        n170 = feedback #17() -> (w361:T1)  [unwired: 1 in]
        n171 = case shown="\"Software\", Default" w361 {
          tunnel: w367 -> [_ w393]
          tunnel: [w384 w385] -> w357
          tunnel: w362 -> [w379 _]
          frame "Software", Default {
            n172 = Compound Arithmetic op=AND(w379, invert "vi/nGenTrig") -> (w383:bool)
            n173 = Compound Arithmetic op=AND("vi/nGenTrig", "TrigIn Simulate") -> (w381:bool)
            n174 = Or(x=w383, y=w381) -> (x .or. y?=w378:bool)
            n175 = call <instrlib>:"Detect Rising Edge.vi"("signal"=w378) -> ("edge detected"=w384:bool)  [unwired: 14 in]
          }
          frame "Data Edge" {
            # "Begins the acquisition after the analog input rises above the trigger level."
            n176 = Unbundle By Name(w393) -> ("Older Data"=w391:u64, "Newer Data"=w389:u64)
            n177 = feedback-in #18("Trigger Level") -> ()
            n178 = feedback #18() -> (w387:i16)  [unwired: 1 in]
            n179 = feedback-in #19(w391) -> ()
            n180 = feedback #19() -> (w386:u64)  [unwired: 1 in]
            n181 = feedback-in #20(w389) -> ()
            n182 = feedback #20() -> (w388:u64)  [unwired: 1 in]
            n183 = call "Data Edge Trigger 8 Samples.vi"("Trigger Level"=w387, "Newer Data In"=w388, "Older Data In"=w386) -> ("Trigger"=w392:bool)  [unwired: 8 in]
            n184 = feedback-in #21(w392) -> ()
            n185 = feedback #21() -> (w385:bool)  [unwired: 1 in]
          }
        }
        n186 = disable-structure shown="Disabled" {
          disable-tunnel: w357 -> [w374 w375]
          disable-tunnel: [w370 w375] -> w356
          frame Disabled {
            n187 = xnode "FPGA I/O Node"() -> ("PXI_Trig0"=w373:bool)  [unwired: 1 in, 1 out]
            n188 = feedback #22() -> (w370:bool)  [unwired: 1 in]
            n189 = call <instrlib>:"Synchronous Latch.vi"("clear"=w370, "set"=w374) -> ("out"=w372:bool)  [unwired: 9 in]
            n190 = And(x=w372, y=w373) -> (x .and. y?=w371:bool)
            n191 = feedback-in #22(w371) -> ()
          }
          frame Enabled {
          }
        }
        n192 = case shown="True" w357 {
          selector: w357 -> [_ w377]
          frame False {
          }
          frame True {
            n193 = xnode ("FIFO Method Node")("Element"=w377, "Timeout"=0) -> ()  [unwired: 1 in, 2 out]
          }
        }
        n194 = Select(t=Aquire_State."Hold Aquire" ("Acquire State"), s=w356, f=Aquire_State."Wait for Trigger") -> (s? t:f=w364:T3)
      }
      frame "Hold Aquire" {
        n195 = xnode "FPGA I/O Node"() -> ("PXI_Trig0"=w399:bool)  [unwired: 1 in, 1 out]
        n196 = feedback #23(TRUE) -> (w395:bool)
        n197 = Not(x=w395) -> (.not. x?=w397:bool)
        n198 = call <instrlib>:"Synchronous Latch.vi"("clear"=w397, "set"=w399) -> ("out"=w398:bool)  [unwired: 9 in]
        n199 = case shown="False" w398 {
          tunnel: w404 -> [w410 w412]
          tunnel: [w410 w411] -> w402
          frame False {
          }
          frame True {
            n200 = Increment(x=w412) -> (x+1=w411:u16)
          }
        }
        n201 = Greater?(x=w403, y=w402) -> (0:w396:bool)
        n202 = feedback-in #23(w396) -> ()
        n203 = Select(t=Aquire_State."Hold Aquire" ("Acquire State"), s=w395, f=Aquire_State."Acquire" ("Acquire State")) -> (s? t:f=w408:T3)
        n204 = case shown="True" w395 {
          tunnel: [u16 0 w414] -> w405
          tunnel: w402 -> [_ w414]
          frame False {
          }
          frame True {
          }
        }
      }
      frame "Acquire" {
        # "Monitor for any  FIFO timeouts"
        # "While in this state, data is pushed into a DMA FIFO until the desired number of samples per record have been acquired."
        n205 = xnode ("FIFO Method Node")("Element"=w426, "Timeout"=0) -> ("Timed Out?"=w421:bool)  [unwired: 1 in, 1 out]
        n206 = Increment(x=w431) -> (x+1=w417:u16)
        n207 = Less?(x=w417, y=w427) -> (x < y?=w415:bool)
        n208 = feedback #24(FALSE) -> (w422:bool)
        n209 = Or(x=w422, y=w421) -> (x .or. y?=w423:bool)
        "TS FIFO In Overflow?" <- w423
        n210 = feedback-in #24(w423) -> ()
        n211 = Select(t=Aquire_State."Acquire" ("Acquire State"), s=w415, f=Aquire_State."WaitForWaveCompletion" ("Acquire State")) -> (s? t:f=w430:T3)
        n212 = case shown="True" w415 {
          tunnel: w417 -> [_ w433]
          tunnel: [u16 0 w433] -> w416
          frame False {
          }
          frame True {
          }
        }
      }
      frame "WaitForWaveCompletion" {
        n213 = local read "WaitForWave\nCompletion"() -> (w434:u16)
        n214 = Increment(x=w440) -> (x+1=w438:u16)
        n215 = Greater?(x=w434, y=w438) -> (0:w437:bool)
        n216 = Select(t=Aquire_State."WaitForWaveCompletion" ("Acquire State"), s=w437, f=Aquire_State."CheckAvg" ("Acquire State")) -> (s? t:f=w444:T3)
        n217 = case shown="True" w437 {
          tunnel: [u16 0 w447] -> w441
          tunnel: w438 -> [_ w447]
          frame False {
          }
          frame True {
          }
        }
      }
      frame "CheckAvg" {
        n218 = Increment(x=w451) -> (x+1=w449:u16)
        n219 = Greater?(x=w450, y=w449) -> (0:w448:bool)
        n220 = case shown="True" w448 {
          selector: w448 -> [_ w459]
          frame False {
          }
          frame True {
            n221 = xnode ("FIFO Method Node")("Element"=w459, "Timeout"=0) -> ()  [unwired: 1 in, 2 out]
          }
        }
        n222 = Select(t=Aquire_State."Hold Aquire" ("Acquire State"), s=w448, f=Aquire_State."Idle") -> (s? t:f=w455:T3)
      }
    }
  }
  n223 = while "Configuration Loop" {
    stop <- FALSE stop-if-true
    # "After the NI 5772 is powered on, the CLIP core provides the module with a default configuration. This loop updates the host VI to the status of the NI 5772 through the Initalization Done Signal. Additionally, this loop configures the Sample clock selection for the NI 5772. Refer to the Clock Select (Host).vi Host VI for more information about how this example configures the clock."
    n224 = xnode "FPGA I/O Node"("IO Module\\User Command"="User Command", "IO Module\\User Data 0"="User Data 0", "IO Module\\User Data 1"="User Data 1", "IO Module\\User Command Commit"="User Command Commit") -> ("IO Module\\User Command Idle"=→"User Command Idle":bool, "IO Module\\User Command Status"=→"User Command Status":u8, "IO Module\\PLL Locked"=→"PLL Locked":bool, "IO Module\\User Error"=w467:u8, "IO Module\\Initialization Done"=→"Configured?":bool)  [unwired: 9 in, 9 out]
    n225 = Not Equal To 0?(x=w467) -> (x != 0?=→"User Error":bool)
  }
  n226 = while "Data Validation/Calculation Loop" {
    stop <- FALSE stop-if-true
    n227 = Scale By Power Of 2(n="AvgCount_powerOf2", x=1 ("Timeout")) -> (x*2^n=w493:i32)
    n228 = To Unsigned Word Integer(number=w493) -> (unsigned 16bit integer=w490:u16)
    n229 = Multiply(x="Delay (us)", y=sgl 200.0) -> (x*y=w486:u16)
    n230 = Divide(x="WaveSampleCount", y="Wave Sampling Rate") -> (x/y=w477:sgl)
    n231 = In Range and Coerce(upper limit=u16 65535, x=w486, lower limit=u16 1) -> (coerced(x)=w478:u16)  [unwired: 1 out]
    "Delay after Trig [cycles]" <- w478
    n232 = In Range and Coerce(upper limit=u16 65535, x=w490, lower limit=u16 1) -> (coerced(x)=→"AvgCount":u16)  [unwired: 1 out]
    n233 = Multiply(x=w477, y=sgl 200000000.0) -> (x*y=w474:sgl)
    n234 = Add(x="Samples Per Trigger", y=w478) -> (x+y=w475:u16)
    n235 = Subtract(x=w474, y=w475) -> (x-y=→"WaitForWave\nCompletion":u16)
    n236 = call "Loop Timer"("Count(uSec)"=u32 100 ("Count(mSec)")) -> ()  [unwired: 1 out]
  }
  n237 = while "TrigOut Loop" {
    stop <- FALSE stop-if-true
    n238 = xnode ("FIFO Method Node")("Timeout"=0) -> ("Element"=w496:bool)  [unwired: 1 in, 2 out]
    n239 = case shown="True" w496 {
      frame False {
      }
      frame True {
        n240 = flat-sequence {
          frame #0 {
            n241 = xnode "FPGA I/O Node"("PXI_Trig1"=TRUE) -> ()  [unwired: 1 in, 1 out]
          }
          frame #1 {
            n242 = call "Wait"("Count(Ticks)"=u32 20 ("Count(uSec)")) -> ()  [unwired: 1 out]
          }
          frame #2 {
            n243 = xnode "FPGA I/O Node"("PXI_Trig1"=FALSE) -> ()  [unwired: 1 in, 1 out]
          }
        }
      }
    }
  }
  n244 = node-c288() -> (w11:T4)  [unwired: 1 in]
  n245 = timed-loop "Trigger In Loop" {
    timing: w11 -> [_]
    timing-out: [_] -> w10
    stop <- FALSE stop-if-true
    # "Triggering is handeled in the 40MHz Loop to remove the signal Jitter and false triggers"
    n246 = xnode "FPGA I/O Node"() -> ("IO Module\\Asynchronous Trigger Input"=w507:bool)  [unwired: 1 in, 1 out]
    n247 = call <instrlib>:"Detect Rising Edge.vi"("signal"=w507) -> ("edge detected"=w504:bool)  [unwired: 14 in]
    n248 = xnode ("FIFO Method Node")("Element"=w507, "Timeout"=0) -> ()  [unwired: 1 in, 2 out]
    n249 = call-poly <instrlib>:"Count Up.vi"("increment"=w504, "reset"="Clear Count") -> ("count out"=→"Trig Count":u64)  [unwired: 13 in]
  }
  n250 = node-c288(w10) -> ()
  n251 = node-c288(w15) -> ()
  n252 = node-c288(w7) -> ()
